vi "readAPDSerial.vi"(8 "Error In":errorcluster) -> (0 "Error Out":errorcluster, 3 "output cluster":T1)   [LabVIEW 2020]
uses:
  <vilib>/Utility/config.llb/Read Key (String).vi
  <vilib>/Utility/config.llb/NI_LVConfig.lvlib
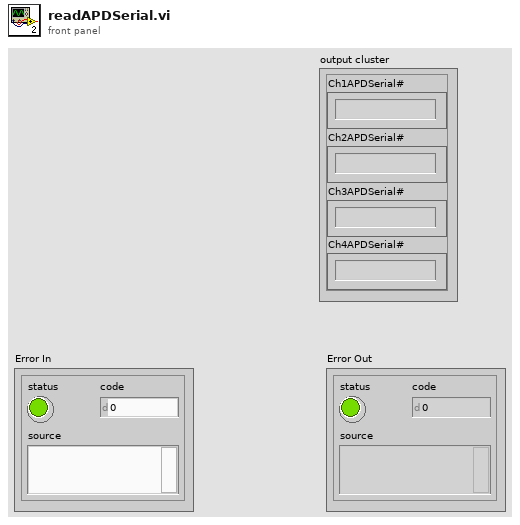
[diagram p1: front panel]
types:
  T1 = cluster{"Ch1APDSerial#":string, "Ch2APDSerial#":string, "Ch3APDSerial#":string, "Ch4APDSerial#":string}
  T2 = typedef "NI_LVConfig.lvlib/Config Data RefNum.ctl" = refnum<k1>
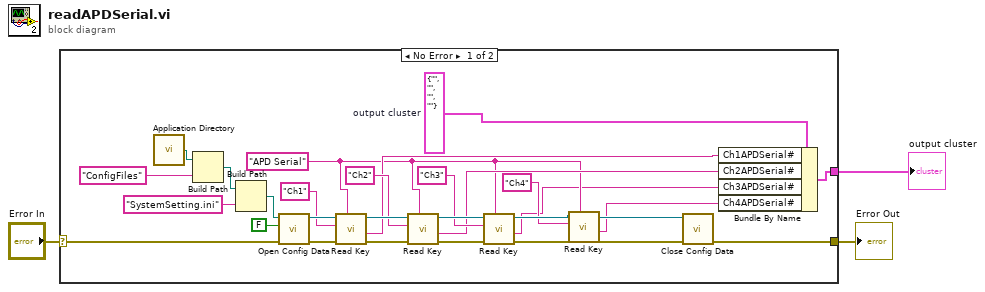
[diagram p0: block diagram]
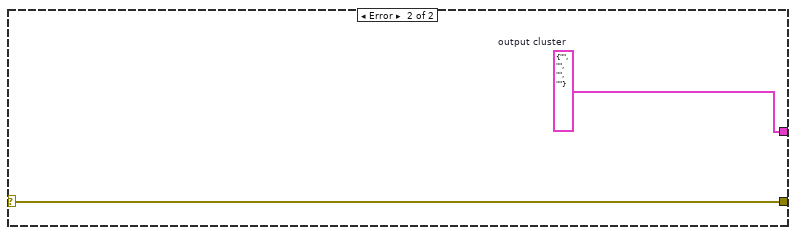
[diagram p2: hidden frame]
diagram:
  n1 = case shown="No Error" "Error In" {
    selector: "Error In" -> [w25 w33]
    tunnel: [w14 w33] -> w2
    tunnel: [w11 w32] -> w1
    frame No Error {
      w10 = T1 {"Ch1APDSerial#"="", "Ch2APDSerial#"="", "Ch3APDSerial#"="", "Ch4APDSerial#"=""}  # output cluster
      w6 = "APD Serial" ("section")
      n2 = call <vilib>:"Application Directory.vi"() -> ("Application Directory"=w31:path)
      n3 = Build Path(base path=w31, name or relative path="ConfigFiles") -> (appended path=w29:path)
      n4 = Build Path(base path=w29, name or relative path="SystemSetting.ini") -> (appended path=w27:path)
      n5 = call <vilib>:"Open Config Data.vi"("error in (no error)"=w25, "create file if necessary (T)"=FALSE, "configuration file path"=w27) -> ("error out"=w23:errorcluster, "refnum"=w24:T2)  [unwired: 6 in, 1 out]
      n6 = call-poly <vilib>:"Read Key.vi"("section"=w6, "error in (no error)"=w23, "key"="Ch1", "refnum"=w24) -> ("error out"=w20:errorcluster, "value"=w13:string, "refnum out"=w21:T2)  [unwired: 4 in, 1 out]
      n7 = call-poly <vilib>:"Read Key.vi"("section"=w6, "error in (no error)"=w20, "key"="Ch2", "refnum"=w21) -> ("error out"=w17:errorcluster, "value"=w12:string, "refnum out"=w18:T2)  [unwired: 4 in, 1 out]
      n8 = call-poly <vilib>:"Read Key.vi"("section"=w6, "error in (no error)"=w17, "key"="Ch3", "refnum"=w18) -> ("error out"=w15:errorcluster, "value"=w5:string, "refnum out"=w9:T2)  [unwired: 4 in, 1 out]
      n9 = call-poly <vilib>:"Read Key.vi"("section"=w6, "key"="Ch4", "refnum"=w9) -> ("value"=w4:string, "refnum out"=w8:T2)  [unwired: 5 in, 2 out]
      n10 = call <vilib>:"Close Config Data.vi"("error in (no error)"=w15, "refnum"=w8) -> ("error out"=w14:errorcluster)  [unwired: 8 in, 1 out]
      n11 = Bundle By Name(cluster=w10, "Ch1APDSerial#"=w13, "Ch2APDSerial#"=w12, "Ch3APDSerial#"=w5, "Ch4APDSerial#"=w4) -> (w11:T1)
    }
    frame Error {
      w32 = T1 {"Ch1APDSerial#"="", "Ch2APDSerial#"="", "Ch3APDSerial#"="", "Ch4APDSerial#"=""}  # output cluster
    }
  }
  "Error Out" <- w2
  "output cluster" <- w1
